vi "Defer Vi.vi"(8 "error in (no error)":errorcluster, 10 "Defer Updates?":bool, 11 "Main Panel in":refnum<class "Main Panel.lvclass">) -> (0 "error out":errorcluster, 3 "Main Panel out":refnum<class "Main Panel.lvclass">)   [LabVIEW 2018, in "Main Panel.lvlib" / "Main Panel.lvclass"]
uses:
  Main Panel.lvclass
  Main Panel.lvclass/Main Panel.ctl
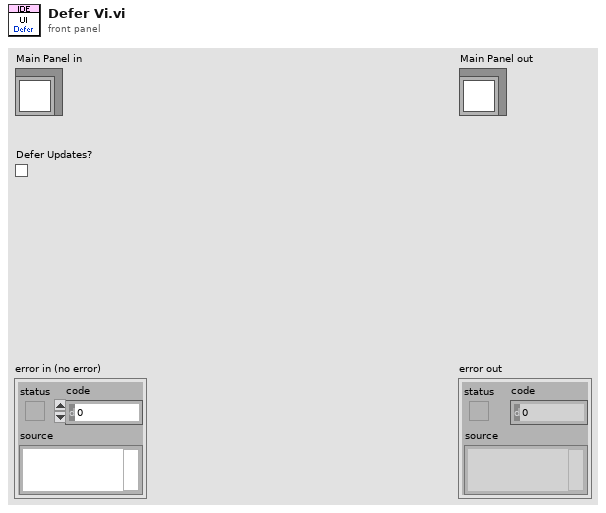
[diagram p1: front panel]
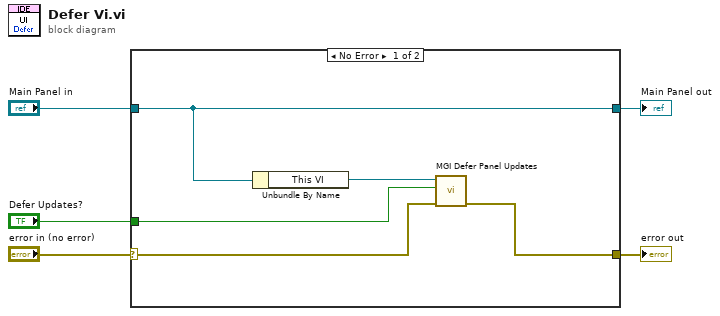
[diagram p0: block diagram]
diagram:
  n1 = case shown="No Error" "error in (no error)" {
    selector: "error in (no error)" -> [w8 w12]
    tunnel: [w7 w12] -> w4
    tunnel: [w10 w11] -> w2
    tunnel: "Main Panel in" -> [w10 w11]
    tunnel: "Defer Updates?" -> [w6 _]
    frame No Error {
      n2 = Unbundle By Name(w10) -> ("This VI"=w9:refnum<vi>)
      n3 = call <userlib>:"MGI Defer Panel Updates.vi"("Error In"=w8, "Defer Updates?"=w6, "VI Reference (Caller)"=w9) -> ("Error Out"=w7:errorcluster)  [unwired: 8 in]
    }
    frame Error {
    }
  }
  "error out" <- w4
  "Main Panel out" <- w2
